vi "Falling Edge Detect.vi"(1 "Input":bool) -> (0 "Output":bool)   [LabVIEW 2013]
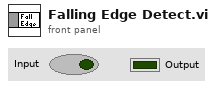
[diagram p1: front panel]
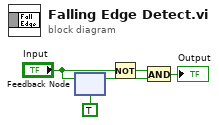
[diagram p0: block diagram]
diagram:
  n1 = feedback #1(TRUE) -> (w3:bool)
  n2 = feedback-in #1("Input") -> ()
  n3 = Not(x="Input") -> (.not. x?=w2:bool)
  n4 = And(x=w2, y=w3) -> (x .and. y?=→"Output":bool)
